vi "setChannel.vi"(8 "error in (no error)":errorcluster, 10 "AnalogOutput":refnum<class "AnalogOutput.lvclass">, 11 "AoDeviceData in":refnum<class "AoDeviceData.lvclass">) -> (0 "error out":errorcluster, 3 "AoDeviceData out":refnum<class "AoDeviceData.lvclass">)   [LabVIEW 2009, in "DataMappers.lvlib" / "AoDeviceData.lvclass"]
uses:
  AoDeviceData.lvclass
  Hal/Channels/VoltOutput/AnalogOutput.lvclass
  AoDeviceData.lvclass/AoDeviceData.ctl
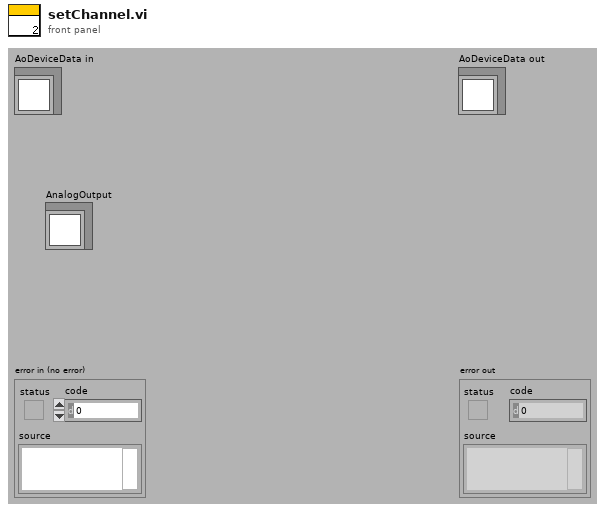
[diagram p1: front panel]
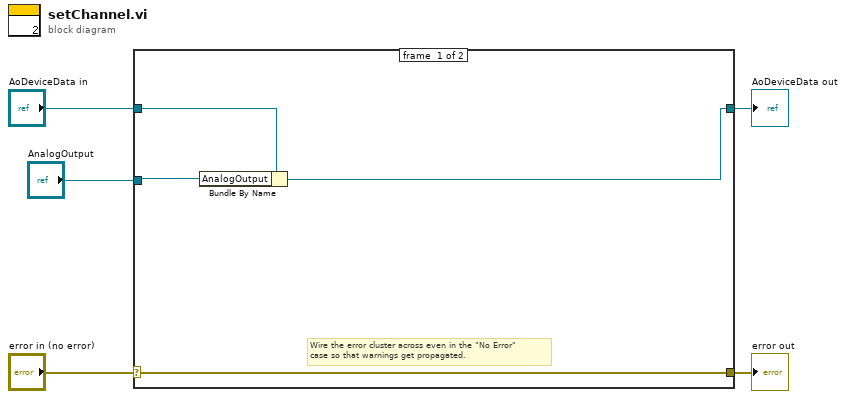
[diagram p0: block diagram]
diagram:
  n1 = case shown="No Error" "error in (no error)" {
    selector: "error in (no error)" -> [w9 w11]
    tunnel: [w9 w11] -> w4
    tunnel: [w6 w10] -> w2
    tunnel: "AoDeviceData in" -> [w7 w10]
    tunnel: "AnalogOutput" -> [w8 _]
    frame #0 {
      # "Wire the error cluster across even in the \"No Error\"\ncase so that warnings get propagated."
      n2 = Bundle By Name(cluster=w7, "AnalogOutput"=w8) -> (w6:refnum<class "AoDeviceData.lvclass">)
    }
    frame #1 {
    }
  }
  "error out" <- w4
  "AoDeviceData out" <- w2
